vi "Normalized spectrum integration.vi"(11 "Frequency domain":cluster{"f0":dbl, "df":dbl, "Magnitude":dbl[]}) -> (1 "NSi 3":dbl, 2 "NSI 2":dbl, 3 "NSI 1":dbl)   [LabVIEW 2019]
panel:
  out "Split magnitude 500 - 1000":dbl[](array[numeric])
  out "split magnitude 250-500":dbl[](array[numeric])
  out "split magnitude 0-250":dbl[](array[numeric])
  out "index of at 500":i32
  out "index of at 250":i32
  out "250 hz tf":bool[](array[boolean])
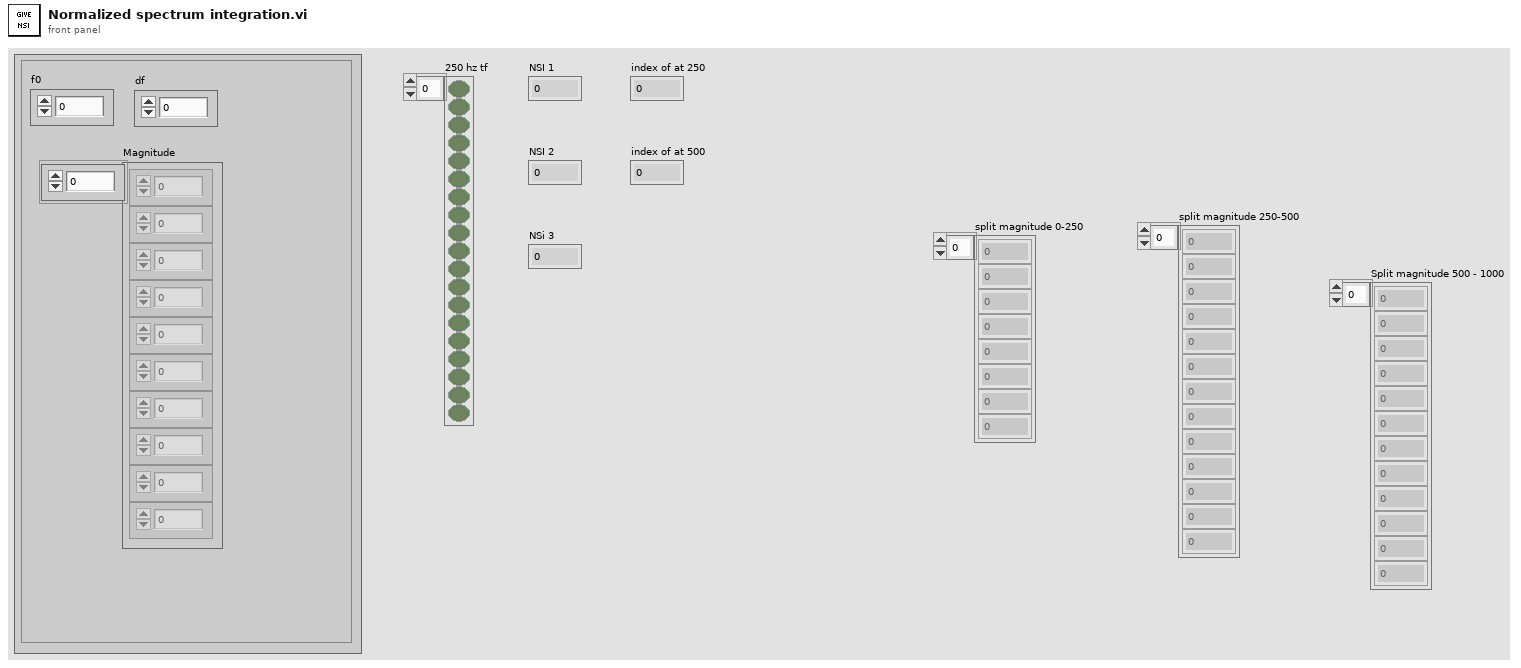
[diagram p1: front panel]
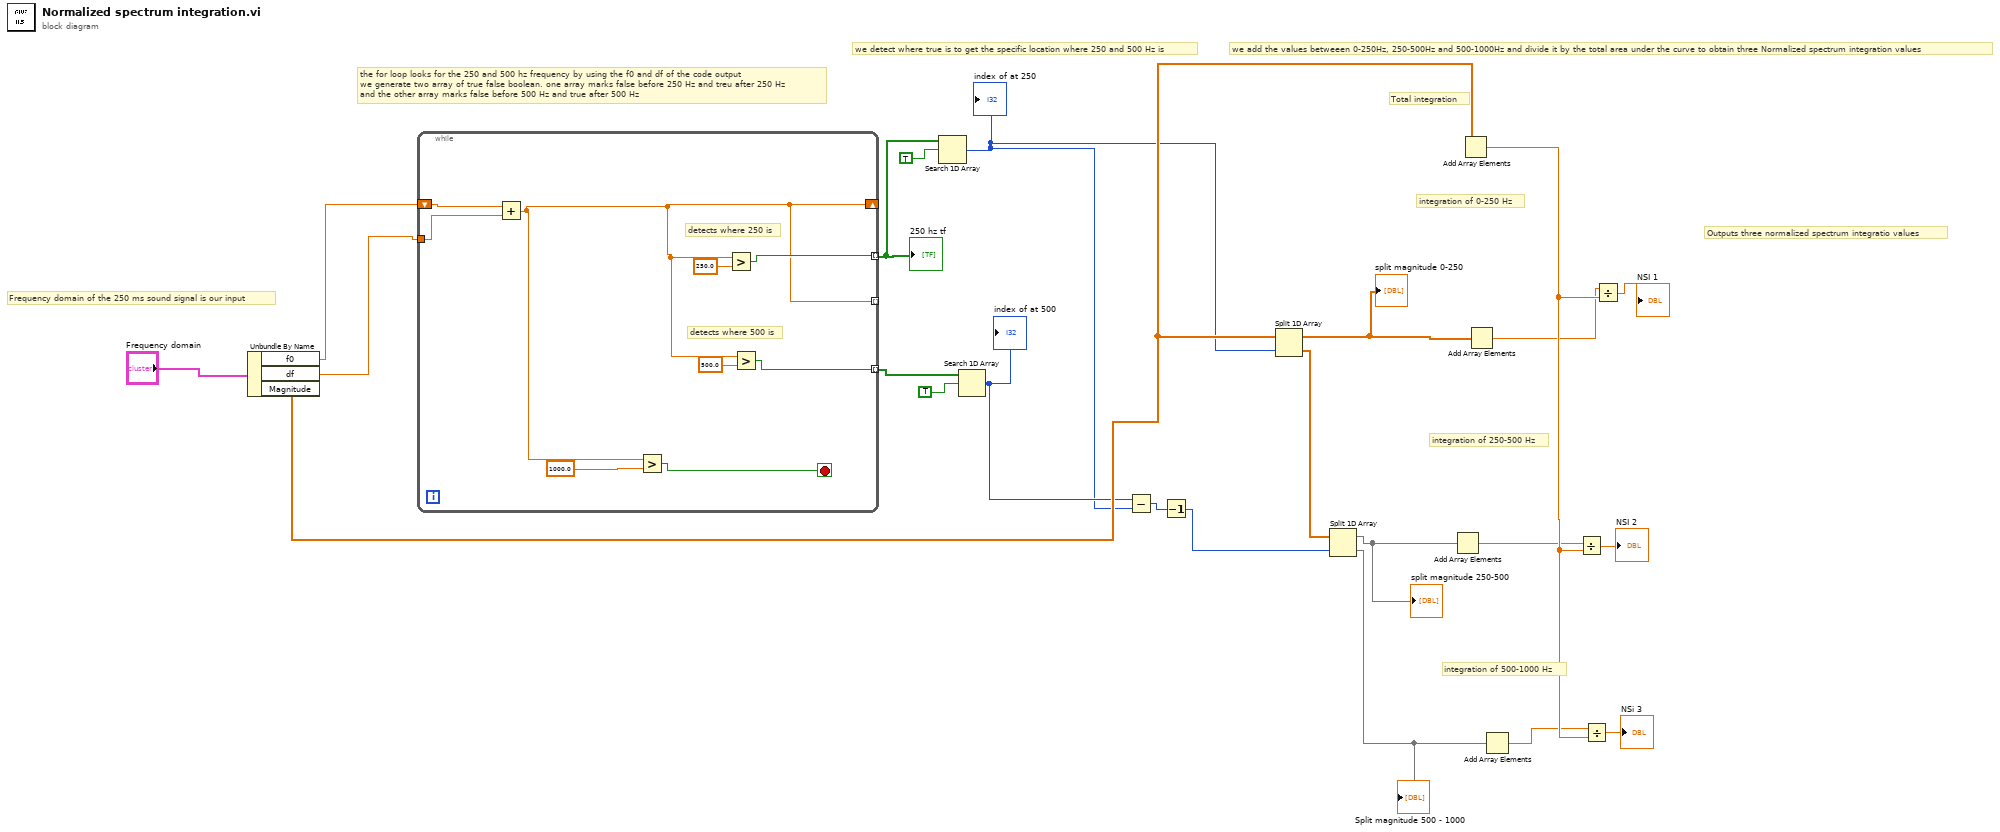
[diagram p0: block diagram]
diagram:
  # "Outputs three normalized spectrum integratio values"
  # "we add the values betweeen 0-250Hz, 250-500Hz and 500-1000Hz and divide it by the total area under the curve to obtain three Normalized spectrum integration values"
  # "we detect where true is to get the specific location where 250 and 500 Hz is"
  # "Frequency domain of the 250 ms sound signal is our input"
  # "the for loop looks for the 250 and 500 hz frequency by using the f0 and df of the code output\nwe generate two array of true false boolean. one array marks false before 250 Hz and treu after 250 Hz \nand the other array marks false before 500 Hz and true after 500 Hz"
  # "Total integration"
  # "integration of 500-1000 Hz"
  # "integration of 250-500 Hz"
  # "integration of 0-250 Hz"
  n1 = Unbundle By Name("Frequency domain") -> ("f0"=w22:dbl, "df"=w21:dbl, "Magnitude"=w10:dbl[])
  n2 = while {
    shift-right: [w25] -> _
    shift-left: w22 -> [w30]
    tunnel: w21 -> [w29]
    tunnel: [w27] -> w20 mode=indexing
    tunnel: [w25] -> _ mode=indexing
    tunnel: [w24] -> w17 mode=indexing
    stop <- w31 stop-if-true
    # "detects where 500 is"
    # "detects where 250 is"
    n3 = Add(x=w30, y=w29) -> (x+y=w25:dbl)
    n4 = Greater?(x=w25, y=1000.0) -> (0:w31:bool)
    n5 = Greater?(x=w25, y=250.0) -> (0:w27:bool)
    n6 = Greater?(x=w25, y=500.0) -> (0:w24:bool)
  }
  "250 hz tf" <- w20
  n7 = Search 1D Array(1D array=w20, element=TRUE) -> (index of element=w4:i32)  [unwired: 1 in]
  "index of at 250" <- w4
  n8 = Search 1D Array(1D array=w17, element=TRUE) -> (index of element=w8:i32)  [unwired: 1 in]
  "index of at 500" <- w8
  n9 = Subtract(x=w8, y=w4) -> (x-y=w9:i32)
  n10 = Decrement(x=w9) -> (x-1=w7:i32)
  n11 = Split 1D Array(array=w10, index=w4) -> (first subarray=w2:dbl[], second subarray=w1:dbl[])
  "split magnitude 0-250" <- w2
  n12 = Split 1D Array(array=w1, index=w7) -> (first subarray=w3:dbl[], second subarray=w13:dbl[])
  "split magnitude 250-500" <- w3
  "Split magnitude 500 - 1000" <- w13
  n13 = Add Array Elements(numeric array=w3) -> (sum=w14:dbl)
  n14 = Add Array Elements(numeric array=w10) -> (sum=w16:dbl)
  n15 = Add Array Elements(numeric array=w2) -> (sum=w11:dbl)
  n16 = Add Array Elements(numeric array=w13) -> (sum=w15:dbl)
  n17 = Divide(x=w14, y=w16) -> (x/y=→"NSI 2":dbl)
  n18 = Divide(x=w15, y=w16) -> (x/y=→"NSi 3":dbl)
  n19 = Divide(x=w11, y=w16) -> (x/y=→"NSI 1":dbl)
